vi "Autofile(SubVI).vi"(8 "error in (no error)":errorcluster, 10 "Filename":string, 11 "File Directory":path) -> (0 "error out":errorcluster, 2 "Output Directory":path, 3 "Byte Stream File out":refnum<file>)   [LabVIEW 2018]
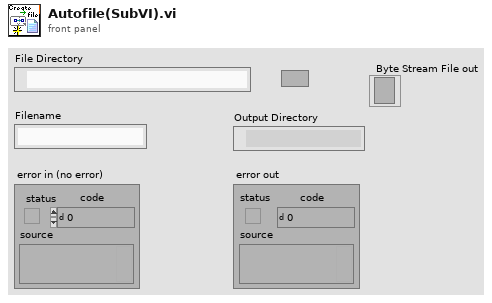
[diagram p1: front panel]
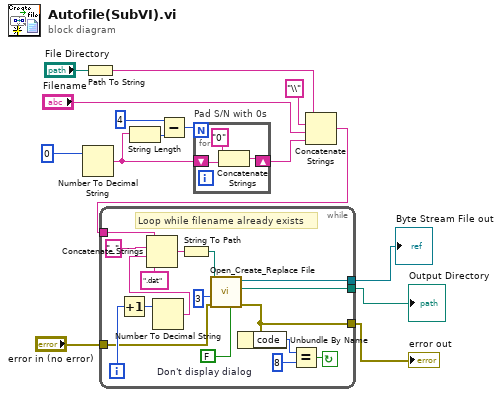
[diagram p0: block diagram]
diagram:
  n1 = Number To Decimal String(number=u16 0 ("Serial Number")) -> (decimal integer string=w2:string)  [unwired: 1 in]
  n2 = Path To String(path="File Directory") -> (string=w5:string)
  n3 = String Length(string=w2) -> (length=w3:i32)
  n4 = Subtract(x=4, y=w3) -> (x-y=w1:i32)
  n5 = for "Pad S/N with 0s" {
    N: w1 -> [_]
    shift-right: [w16] -> w9
    shift-left: w2 -> [w17]
    n6 = Concatenate Strings("0", w17) -> (w16:string)
  }
  n7 = Concatenate Strings(w5, "\\", "Filename", w9) -> (w7:string)
  n8 = while {
    tunnel: [w28] -> w10
    tunnel: w7 -> [w29]
    tunnel: [w24] -> w15
    tunnel: [w20] -> w11
    tunnel: "error in (no error)" -> [w19]
    i -> [w34]
    stop <- w23 continue-if-true
    w27 = FALSE  # Don't display dialog
    # "Loop while filename already exists"
    n9 = Increment(x=w34) -> (x+1=w35:i32)
    n10 = Number To Decimal String(number=w35) -> (decimal integer string=w26:string)  [unwired: 1 in]
    n11 = Concatenate Strings(w29, "_", w26, ".dat") -> (w32:string)
    n12 = String To Path(string=w32) -> (path=w30:path)
    n13 = call <vilib>:"Open_Create_Replace File.vi"("advisory dialog? (display:T)"=w27, "error in (no error)"=w19, "function (open:0)"=3, "file path"=w30) -> ("error out"=w24:errorcluster, "new file path"=w20:path, "refnum"=w28:refnum<file>)  [unwired: 4 in, 1 out]
    n14 = Unbundle By Name(w24) -> ("code"=w22:i32)
    n15 = Equal?(x=w22, y=8) -> (x = y?=w23:bool)
  }
  "Output Directory" <- w11
  "Byte Stream File out" <- w10
  "error out" <- w15
